vi "test DOCTYPE Declaration 001.vi"(8 "error in (no error)":errorcluster, 11 "TestCase in":refnum<class "EasyXMLTest.lvclass">) -> (0 "error out":errorcluster, 3 "TestCase out":refnum<class "EasyXMLTest.lvclass">)   [LabVIEW 2013, in "EasyXMLTest.lvclass"]
doc: "Verify that error in is not overwritten"
uses:
  EasyXMLTest.lvclass
panel:
  out "Produced Data":variant
  out "Input Data":variant
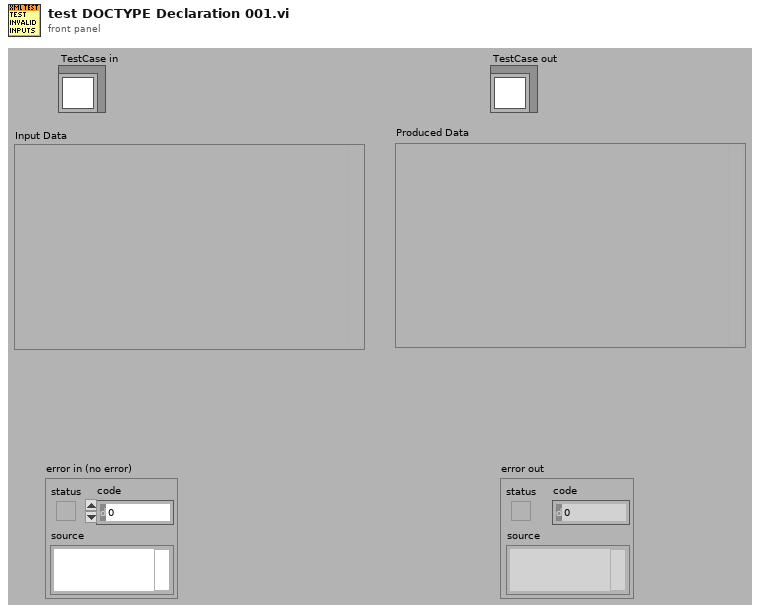
[diagram p1: front panel]
types:
  T1 = cluster{"#attributes":cluster{"xmlns":string, "xml:lang":string, "lang":string}, "html":string}
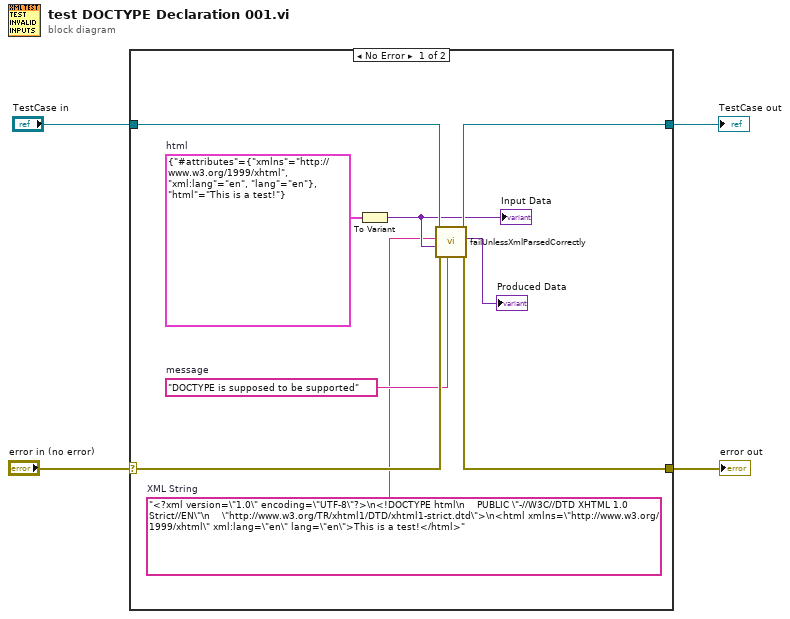
[diagram p0: block diagram]
diagram:
  n1 = case shown="No Error" "error in (no error)" {
    selector: "error in (no error)" -> [w9 w15]
    tunnel: [w8 w15] -> w2
    tunnel: [w12 w14] -> w1
    tunnel: "TestCase in" -> [w13 w14]
    frame No Error {
      w5 = "<?xml version=\"1.0\" encoding=\"UTF-8\"?>\n<!DOCTYPE html\n    PUBLIC \"-//W3C//DTD XHTML 1.0 Strict//EN\"\n    \"http://www.w3.org/TR/xhtml1/DTD/xhtml1-strict.dtd\">\n<html xmlns=\"http://www.w3.org/1999/xhtml\" xml:lang=\"en\" lang=\"en\">This is a test!</html>"  # XML String
      w10 = T1 {"#attributes"={"xmlns"="http://www.w3.org/1999/xhtml", "xml:lang"="en", "lang"="en"}, "html"="This is a test!"}  # html
      w7 = "DOCTYPE is supposed to be supported"  # message
      n2 = To Variant(anything=w10) -> (Variant=w6:variant)
      "Input Data" <- w6
      n3 = call "failUnlessXmlParsedCorrectly.vi"("message (\"\")"=w7, "error in"=w9, "Expected Data"=w6, "XML String"=w5, "reference in"=w13) -> ("error out"=w8:errorcluster, "Produced Data"=→"Produced Data":variant, "reference in"=w12:refnum<class "EasyXMLTest.lvclass">)  [unwired: 4 in]
    }
    frame Error {
    }
  }
  "error out" <- w2
  "TestCase out" <- w1
